vi "Send Command.vi"(8 "Error In":errorcluster, 9 "ARGS":u8[](array[numeric]), 10 "CMD":u16, 11 "LINX Device Config":T1) -> (0 "Error Out":errorcluster, 1 "Status":u8, 2 "Response":u8[](array[numeric]), 3 "LINX Device Config":T1)   [LabVIEW 2011, in "LVH-LINX.lvlib" / "Device.lvlib"]
doc: "Send a packet to the LINX device and return the LINX device response packet."
uses:
  Device.lvlib
  Type Defs/LINX Device Config.ctl
  Type Defs/Interface.ctl
  Type Defs/TCP Config.ctl
  Type Defs/Device Family.ctl
  Type Defs/Error Type.ctl
  LVH-LINX.lvlib
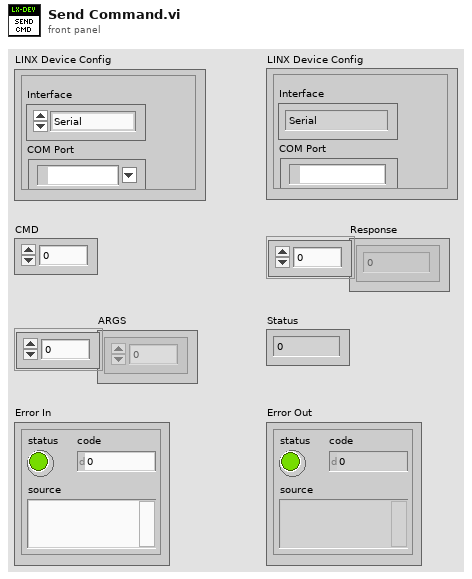
[diagram p1: front panel]
types:
  T1 = typedef "LVH-LINX.lvlib/Device.lvlib/LINX Device Config.ctl" = cluster{"Interface":T2, "COM Port":refnum<visa-resource-name>, "TCP Configuration":T3, "Device Family":T4, "Device ID":u8, "Device Name":string, "TCP Ref":refnum<k5>}
  T2 = typedef "LVH-LINX.lvlib/Interface.ctl" = enum16{"Serial", "TCP"}
  T3 = typedef "LVH-LINX.lvlib/Device.lvlib/TCP Config.ctl" = cluster{"IP Address":string, "Port":u16}
  T4 = typedef "LVH-LINX.lvlib/Device Family.ctl" = enum8{"National Instruments", "Digilent", "Arduino"}
  T5 = typedef "LVH-LINX.lvlib/Error Type.ctl" = enum16{"Unknown", "Timeout", "Corrupt Return Packet", "Unable To Connect", "Command Not Supported", "Channel DNE"}
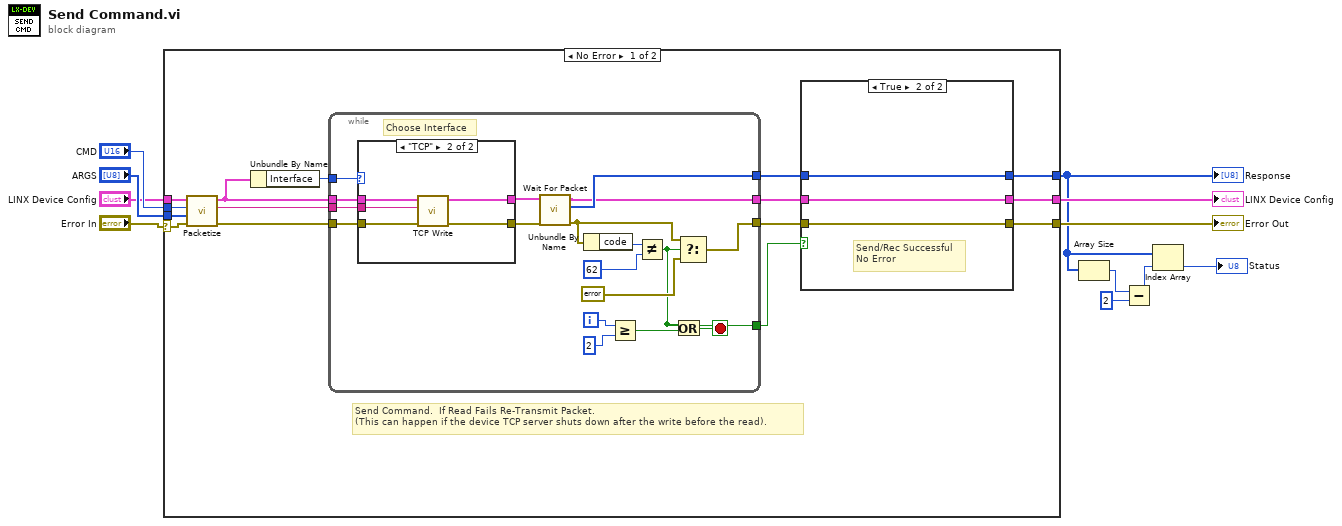
[diagram p0: block diagram]
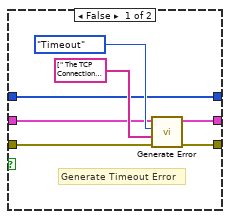
[diagram p2: hidden frame]
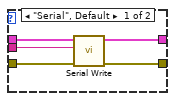
[diagram p3: hidden frame]
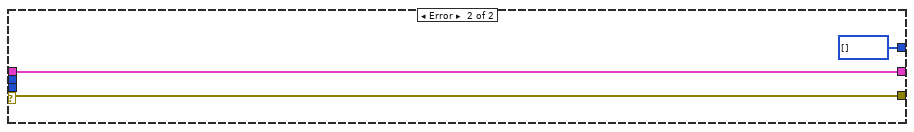
[diagram p4: hidden frame]
diagram:
  n1 = case shown="No Error" "Error In" {
    selector: "Error In" -> [w12 w65]
    tunnel: "ARGS" -> [w24 _]
    tunnel: "CMD" -> [w23 _]
    tunnel: "LINX Device Config" -> [w20 w67]
    tunnel: [w18 w67] -> w8
    tunnel: [w17 w65] -> w7
    tunnel: [w14 u8[] [] ("Packet")] -> w5
    frame No Error {
      # "Send Command.  If Read Fails Re-Transmit Packet.\n(This can happen if the device TCP server shuts down after the write before the read)."
      n2 = call "Packetize.vi"("Error In"=w12, "ARGS"=w24, "CMD"=w23, "LINX Device Config"=w20) -> ("Error Out"=w26:errorcluster, "Packet"=w25:string, "LINX Decice Config"=w22:T1)  [unwired: 5 in]
      n3 = Unbundle By Name(w22) -> ("Interface"=w21:T2)
      n4 = while {
        tunnel: w26 -> [w54]
        tunnel: w25 -> [w53]
        tunnel: w22 -> [w52]
        tunnel: w21 -> [w51]
        tunnel: [w50] -> w13
        tunnel: [w37] -> w16
        tunnel: [w47] -> w15
        tunnel: [w39] -> w19
        i -> [w43]
        stop <- w40 stop-if-true
        # "Choose Interface"
        n5 = case shown="\"TCP\"" w51 {
          tunnel: w52 -> [w58 w62]
          tunnel: w54 -> [w59 w63]
          tunnel: [w55 w60] -> w49
          tunnel: [w56 w61] -> w48
          tunnel: w53 -> [w57 w64]
          frame "Serial", Default {
            n6 = call "Serial Write.vi"("Error In"=w59, "Data"=w57, "LINX Device Config"=w58) -> ("Error Out"=w55:errorcluster, "LINX Device Config"=w56:T1)  [unwired: 7 in]
          }
          frame "TCP" {
            n7 = call "TCP Write.vi"("Error In"=w63, "Packet"=w64, "LINX Decice Config"=w62) -> ("Error Out"=w60:errorcluster, "LINX Decice Config"=w61:T1)  [unwired: 7 in]
          }
        }
        n8 = call "Wait For Packet.vi"("Error In"=w49, "LINX Device Config"=w48) -> ("Error Out"=w38:errorcluster, "Packet"=w50:u8[], "LINX Device Config"=w47:T1)  [unwired: 7 in]
        n9 = Unbundle By Name(w38) -> ("code"=w46:i32)
        n10 = Greater Or Equal?(x=w43, y=2) -> (x >= y?=w41:bool)
        n11 = Not Equal?(x=w46, y=62) -> (x != y?=w39:bool)
        n12 = Or(x=w39, y=w41) -> (x .or. y?=w40:bool)
        n13 = Select(t=w38, s=w39, f=errorcluster {"status"=FALSE, "code"=0, "source"=""}) -> (s? t:f=w37:errorcluster)
      }
      n14 = case shown="True" w19 {
        tunnel: [w33 w34] -> w17
        tunnel: [w30 w35] -> w18
        tunnel: w16 -> [w29 w34]
        tunnel: w15 -> [w28 w35]
        tunnel: [w27 w36] -> w14
        tunnel: w13 -> [w27 w36]
        frame False {
          # "Generate Timeout Error"
          n15 = call "Generate Error.vi"("Error In"=w29, "Arguments"=string[] [" The TCP Connection Was Refused."], "Error Type"=Error_Type."Timeout", "LINX Device Config"=w28) -> ("Error Out"=w33:errorcluster, "LINX Device Config"=w30:T1)  [unwired: 6 in]
        }
        frame True {
          # "Send/Rec Successful\nNo Error"
        }
      }
    }
    frame Error {
    }
  }
  "Error Out" <- w7
  "Response" <- w5
  "LINX Device Config" <- w8
  n16 = Array Size(array=w5) -> (size(s)=w4:i32)
  n17 = Subtract(x=w4, y=2 ("x")) -> (x-y=w3:i32)
  n18 = Index Array(array=w5, index=w3) -> (element=→"Status":u8)
